vi "Read Type Mask.vi"(8 "Error In":errorcluster, 11 "Known Host In":refnum<class "KnownHost.lvclass">) -> (0 "Error Out":errorcluster, 2 "Type Mask":i32, 3 "Known Host Out":refnum<class "KnownHost.lvclass">)   [LabVIEW 2017, in "Toolkit.lvlib" / "KnownHost.lvclass"]
uses:
  KnownHost.lvclass
  KnownHost.lvclass/KnownHost.ctl
  Toolkit.lvlib
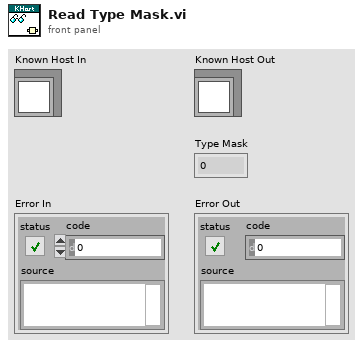
[diagram p1: front panel]
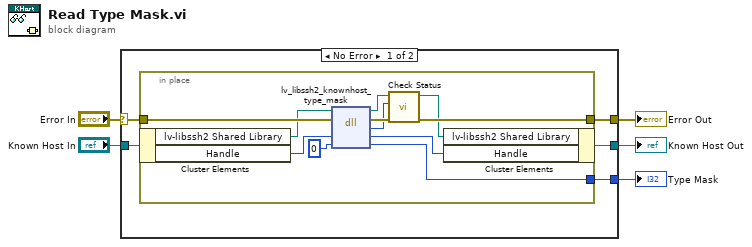
[diagram p0: block diagram]
diagram:
  n1 = case shown="No Error" "Error In" {
    selector: "Error In" -> [w10 w23]
    tunnel: [w9 w23] -> w4
    tunnel: "Known Host In" -> [w8 w22]
    tunnel: [w7 w22] -> w2
    tunnel: [w6 _] -> w1
    frame No Error {
      n2 = in-place {
        in-place-border: w10 -> [w21]
        in-place-border: [w15] -> w9
        in-place-border: [w11] -> w6
        n3 = in-place-cluster #1(w8) -> ("lv-libssh2 Shared Library"=w20:path, "Handle"=w19:u64)
        n4 = dll-call lib="lv-libssh2.*" fn="lv_libssh2_knownhost_type_mask"(path in=w20, error in=w21, "handle"=w19, "type_mask"=0 ("magic")) -> (path out=w14:path, error out=w16:errorcluster, "status"=w12:i32, "handle"=w18:u64, "type_mask"=w11:i32)  [unwired: 1 in]
        n5 = call "Check Status.vi"("Error In"=w16, "Status"=w12, "lv-libssh2 Shared Library In"=w14) -> ("Error Out"=w15:errorcluster, "lv-libssh2 Shared Library Out"=w13:path)  [unwired: 7 in]
        n6 = in-place-cluster #1("lv-libssh2 Shared Library"=w13, "Handle"=w18) -> (w7:refnum<class "KnownHost.lvclass">)
      }
    }
    frame Error {
    }
  }
  "Error Out" <- w4
  "Known Host Out" <- w2
  "Type Mask" <- w1
